vi "SubViTriangulo.vi"() -> ()   [LabVIEW 2018]
panel:
  out "String":string
  out "Menor 0":bool
  out "Area of Triangle":dbl
  in  "Side C":dbl
  in  "Side B":dbl
  in  "Side A":dbl
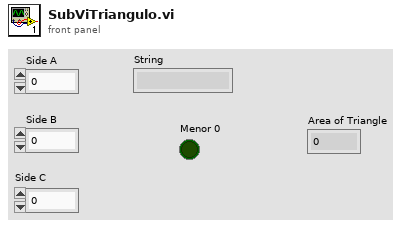
[diagram p1: front panel]
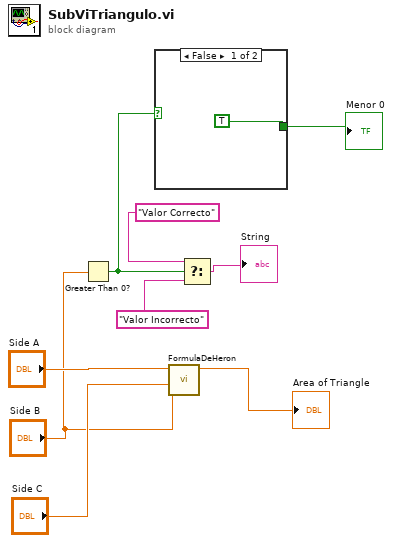
[diagram p0: block diagram]
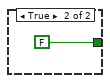
[diagram p2: hidden frame]
diagram:
  n1 = Greater Than 0?(x="Side B") -> (x > 0?=w3:bool)
  n2 = case shown="False" w3 {
    tunnel: [TRUE FALSE] -> w2
    frame False {
    }
    frame True {
    }
  }
  "Menor 0" <- w2
  n3 = call "FormulaDeHeron.vi"("c"="Side C", "b"="Side B", "a"="Side A") -> ("Area Triangulo"=→"Area of Triangle":dbl)  [unwired: 6 in]
  n4 = Select(t="Valor Correcto", s=w3, f="Valor Incorrecto") -> (s? t:f=→"String":string)
